vi "Parse_ReadAnalogIn_2D3.vi"(10 "ReadAnalogIn_Input":string) -> (0 "MIC_2_OUT_DIAG_HIGHRES":dbl, 1 "MIC_1_OUT_DIAG_HIGHRES":dbl, 2 "MIC_2_DIAG_HIGHRES":dbl, 3 "MIC_1_DIAG_HIGHRES":dbl)   [LabVIEW 2015]
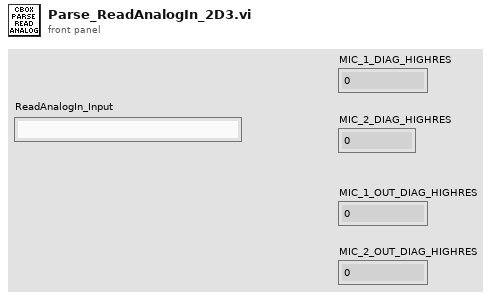
[diagram p1: front panel]
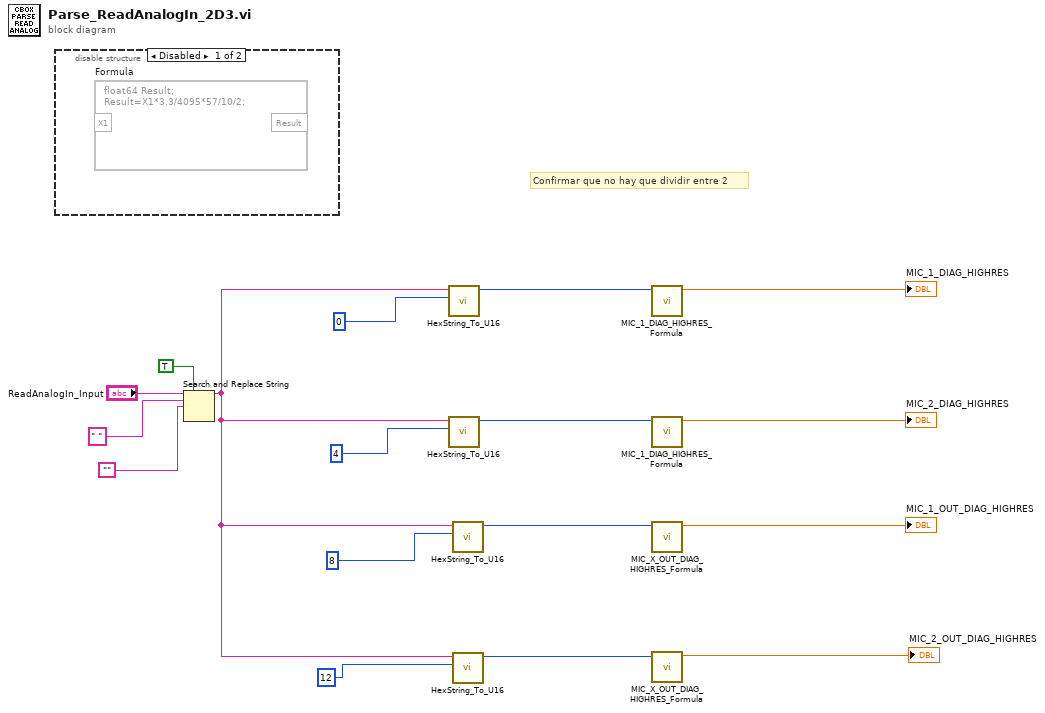
[diagram p0: block diagram]
diagram:
  # "Confirmar que no hay que dividir entre 2"
  n1 = disable-structure shown="Disabled" {
    frame Disabled {
      n2 = formula code="float64 Result;\nResult=X1*3.3/4095*57/10/2;"() -> ()  [unwired: 1 in, 1 out]
    }
    frame Enabled {
    }
  }
  n3 = Search and Replace String(replace all?=TRUE ("replace all? (F)"), input string="ReadAnalogIn_Input", search string=" ", replace string="") -> (result string=w8:string)  [unwired: 4 in, 3 out]
  n4 = call "HexString_To_U16.vi"("Position"=0, "String"=w8) -> ("U16"=w6:u32)  [unwired: 9 in]
  n5 = call "HexString_To_U16.vi"("Position"=4 ("length (rest)"), "String"=w8) -> ("U16"=w4:u32)  [unwired: 9 in]
  n6 = call "HexString_To_U16.vi"("Position"=8 ("length (rest)"), "String"=w8) -> ("U16"=w10:u32)  [unwired: 9 in]
  n7 = call "HexString_To_U16.vi"("Position"=12 ("length (rest)"), "String"=w8) -> ("U16"=w9:u32)  [unwired: 9 in]
  n8 = call "MIC_1_DIAG_HIGHRES_Formula.vi"("Numeric in"=w6) -> ("Numeric out"=→"MIC_1_DIAG_HIGHRES":dbl)  [unwired: 10 in]
  n9 = call "MIC_1_DIAG_HIGHRES_Formula.vi"("Numeric in"=w4) -> ("Numeric out"=→"MIC_2_DIAG_HIGHRES":dbl)  [unwired: 10 in]
  n10 = call "MIC_X_OUT_DIAG_HIGHRES_Formula.vi"("Numeric in"=w10) -> ("Numeric out"=→"MIC_1_OUT_DIAG_HIGHRES":dbl)  [unwired: 10 in]
  n11 = call "MIC_X_OUT_DIAG_HIGHRES_Formula.vi"("Numeric in"=w9) -> ("Numeric out"=→"MIC_2_OUT_DIAG_HIGHRES":dbl)  [unwired: 10 in]
